vi "Test_ARGB_Data_to_Pixel_Data.vi"(8 "error in (no error)":errorcluster, 11 "Test Case In":refnum<class "Image.lvclass">) -> (0 "error out":errorcluster, 3 "Test Case Out":refnum<class "Image.lvclass">)   [LabVIEW 2020, in "g_ar_toolkit.test.lvlib" / "Image.lvclass"]
uses:
  Image.lvclass
  C:/Program Files (x86)/National Instruments/LabVIEW 2020/vi.lib/Astemes/LUnit/Test Case.lvclass
  g_ar_toolkit.image/Image Size (Fixed).ctl
  <vilib>/Astemes/LUnit/Test Case.lvclass/Test Case.ctl
  <vilib>/Astemes/LUnit/Append Pass Result.vi
  <vilib>/Astemes/LUnit/Append Fail Result.vi
  <vilib>/Astemes/LUnit/Describe Comparison.vi
  <vilib>/Astemes/LUnit/Compare Variants.vi
  <vilib>/Astemes/LUnit/Variant to string.vi
  <vilib>/picture/picture.llb/Draw Rectangle.vi
  <vilib>/picture/pictutil.llb/Picture to Pixmap.vi
  <vilib>/Utility/Data Type/Get Type Information.vi
  <vilib>/Utility/LVClass/Get LV Class Name.vi
  Image.lvclass/Image.ctl
  4993e8ee-a06a-463a-9684-69129f64d5ce.vi
  eb111072-ef64-4670-bf69-e7e9452429d1.vi
  g_ar_toolkit.image/g_ar_toolkit.image.lvlib
panel:
  out "new picture":picture
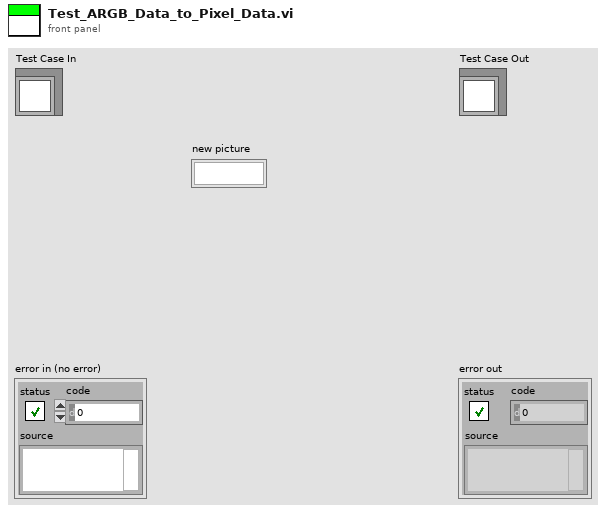
[diagram p1: front panel]
types:
  T1 = typedef "g_ar_toolkit.image.lvlib/Image Size (Fixed).ctl" = cluster{"Width":u16, "Height":u16}
  T2 = typedef "imagedata.ctl" = cluster{"image type":i32, "image depth":i32, "image":u8[], "mask":u8[], "colors":u32[], "Rectangle":cluster{"left":i16, "top":i16, "right":i16, "bottom":i16}}
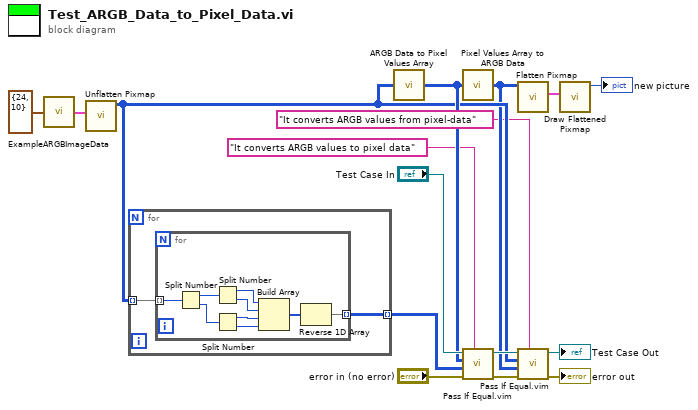
[diagram p0: block diagram]
diagram:
  n1 = call "ExampleARGBImageData.vi"("Image Size"=T1 {"Width"=24, "Height"=10}) -> ("RGB Image Data"=w14:T2)
  n2 = call <vilib>:"Unflatten Pixmap.vi"("image data"=w14) -> ("24-bit pixmap"=w3:u32[][])  [unwired: 4 in, 6 out]
  n3 = for {
    tunnel: w3 -> [w18] mode=indexing
    tunnel: [w17] -> w10 mode=indexing
    n4 = for {
      tunnel: w18 -> [w27] mode=indexing
      tunnel: [w19] -> w17 mode=indexing
      n5 = Split Number(x=w27) -> (hi(x)=w26:u16, lo(x)=w25:u16)
      n6 = Split Number(x=w26) -> (hi(x)=w23:u8, lo(x)=w22:u8)
      n7 = Split Number(x=w25) -> (hi(x)=w21:u8, lo(x)=w20:u8)
      n8 = Build Array(w23, w22, w21, w20) -> (w24:u8[])
      n9 = Reverse 1D Array(array=w24) -> (reversed array=w19:u8[])
    }
  }
  n10 = call "ARGB Data to Pixel Values Array.vi"("ARGB Data"=w3) -> ("Pixel Values"=w9:u8[][][])
  n11 = call "Pixel Values Array to ARGB Data.vi"("Pixel Values"=w9) -> ("ARGB Data"=w2:u32[][])
  n12 = call "Pass If Equal.vim"("Description"="It converts ARGB values to pixel data", "error in (no error)"="error in (no error)", "Actual"=w10, "Expected"=w9, "LUnit Test Case In"="Test Case In") -> ("error out"=w7:errorcluster, "LUnit Test Case Out"=w6:refnum<class "Image.lvclass">)  [unwired: 5 in]
  n13 = call <vilib>:"Flatten Pixmap.vi"("24-bit pixmap"=w2) -> ("image data"=w13:T2)  [unwired: 10 in]
  n14 = call "Pass If Equal.vim"("Description"="It converts ARGB values from pixel-data", "error in (no error)"=w7, "Actual"=w2, "Expected"=w3, "LUnit Test Case In"=w6) -> ("error out"=→"error out":errorcluster, "LUnit Test Case Out"=→"Test Case Out":refnum<class "Image.lvclass">)  [unwired: 5 in]
  n15 = call <vilib>:"Draw Flattened Pixmap.vi"("image data"=w13) -> ("new picture"=→"new picture":picture)  [unwired: 8 in]
